vi "Remote Video 1Hz livestream (TCP SERVER).vi"(1 "Quality":i32=750 min=0 max=1000, 2 "Resolution":T1=1 items=["Low", "Med", "High", "Max."], 3 "TCP/IP port":u16=80, 4 "Camera":T2="Travcam") -> (0 "Error out":errorcluster)   [LabVIEW 2015]
uses:
  Camera enum/Camera enum.ctl
  Camera enum/Camera resolution.ctl
  Globals/CamServer global.vi
panel:
  # "PN 01/09/15"
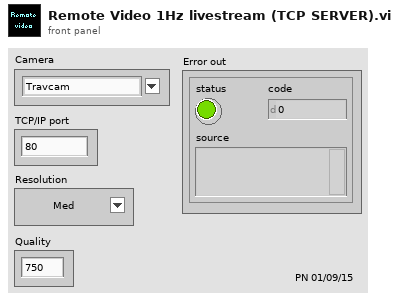
[diagram p1: front panel]
types:
  T1 = typedef "Camera resolution.ctl" = u8
  T2 = typedef "Camera enum.ctl" = string
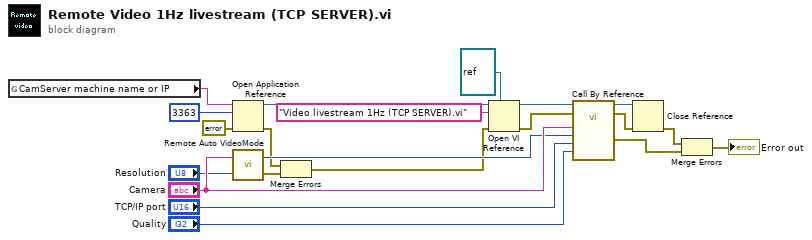
[diagram p0: block diagram]
diagram:
  n1 = global read "CamServer global.vi" "CamServer machine name or IP"() -> (w7:string)
  n2 = Open Application Reference(8:errorcluster {"status"=FALSE, "code"=0, "source"=""} ("error in (no error)"), 10:u16 3363 ("port"), 11:w7) -> (0:w4:errorcluster, 3:w19:refnum<vi>)  [unwired: 1 in]
  n3 = call "Remote Auto VideoMode.vi"("Resolution"="Resolution", "Camera"="Camera") -> ("Error out"=w5:errorcluster, "VideoMode"=w10:u32)
  n4 = Merge Errors(w4, w5) -> (w3:errorcluster)
  n5 = Open VI Reference(type specifier VI Refnum (for type only)=refnum<vi> refnum, application reference (local)=w19, vi path="Video livestream 1Hz (TCP SERVER).vi" ("machine name"), error in (no error)=w3) -> (vi reference=w17:refnum<vi>, error out=w18:errorcluster)  [unwired: 2 in]
  n6 = call-by-ref "?"(reference=w17, error in=w18, "Quality"="Quality", "TCP/IP port"="TCP/IP port", "VideoMode"=w10, "Interface name"="Camera") -> (reference out=w16:refnum<vi>, error out=w15:errorcluster, "Error Out"=w14:errorcluster)
  n7 = Close Reference(reference=w16, error in (no error)=w15) -> (error out=w13:errorcluster)
  n8 = Merge Errors(w13, w14) -> (→"Error out":errorcluster)
